vi "例3.2随机数和表达式节点的使用.vi"() -> ()   [LabVIEW 2012]
panel:
  out "产生的随机数":dbl
  in  "输入":dbl
  out "结果":dbl
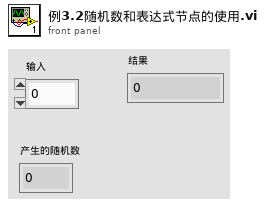
[diagram p1: front panel]
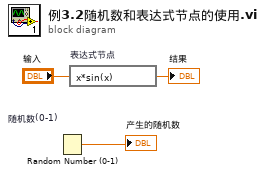
[diagram p0: block diagram]
diagram:
  n1 = Random Number (0-1) "随机数(0-1)"() -> (number: 0 to 1=→"产生的随机数":dbl)
  n2 = expression code="x*sin(x)" "表达式节点"("输入") -> (→"结果":dbl)
